vi "erForceRobotControl.vi"(8 "error in (no error)":errorcluster, 10 "robots":T1[](array[typedef]), 11 "Communication in":refnum<class "Communication.lvclass">) -> (0 "error out":errorcluster, 2 "robotControl":u8[](array[numeric]), 3 "Communication out":refnum<class "Communication.lvclass">)   [LabVIEW 2023, in "Communication.lvclass"]
uses:
  Communication.lvclass
  Convert AI Robot to Robot Command Folder/grSim/grSim Robot Command.ctl
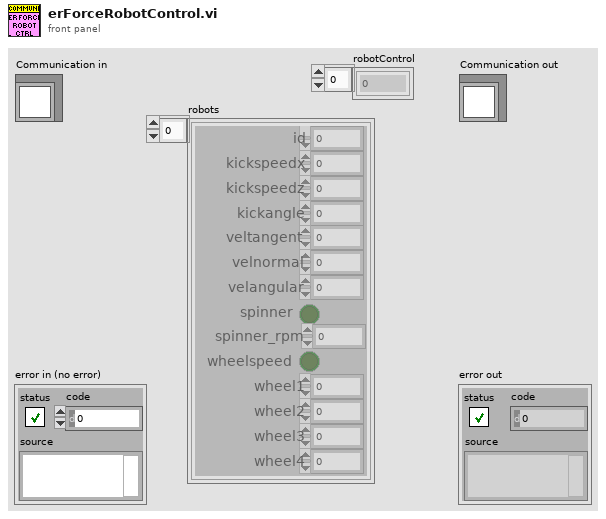
[diagram p1: front panel]
types:
  T1 = typedef "grSim Robot Command.ctl" = cluster{"id":u32, "kickspeedx":sgl, "kickspeedz":sgl, "veltangent":sgl, "velnormal":sgl, "velangular":sgl, "spinner":bool, "wheelspeed":bool, "wheel1":sgl, "wheel2":sgl, "wheel3":sgl, "wheel4":sgl, "kickangle":sgl, "spinner_rpm":sgl}
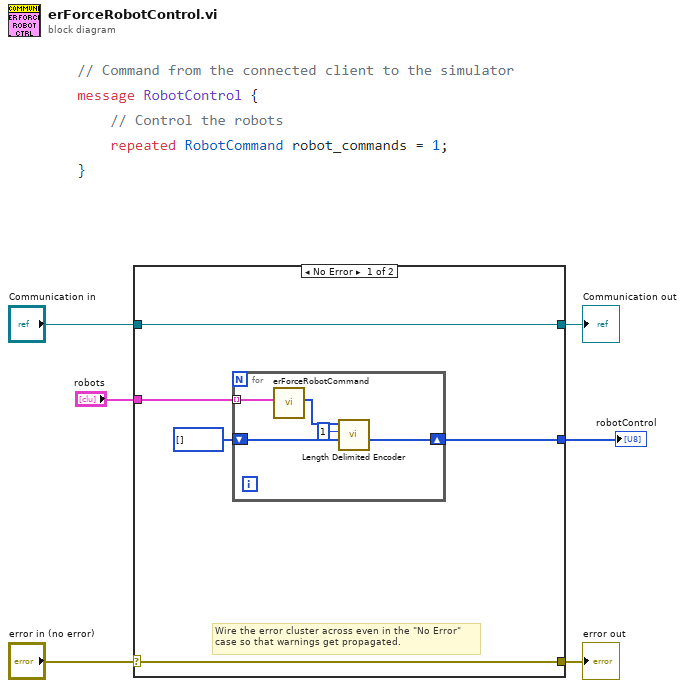
[diagram p0: block diagram]
diagram:
  n1 = case shown="No Error" "error in (no error)" {
    selector: "error in (no error)" -> [w10 w18]
    tunnel: [w10 w18] -> w5
    tunnel: [w11 w17] -> w3
    tunnel: "Communication in" -> [w11 w17]
    tunnel: [w9 _] -> w2
    tunnel: "robots" -> [w8 _]
    frame No Error {
      # "Wire the error cluster across even in the \"No Error\"\ncase so that warnings get propagated."
      n2 = for {
        shift-right: [w15] -> w9
        shift-left: u8[] [] ("Array") -> [w14]
        tunnel: w8 -> [w12] mode=indexing
        n3 = call "erForceRobotCommand.vi"("robot"=w12) -> ("robotCommandArray out"=w16:u8[])  [unwired: 8 in, 2 out]
        n4 = call "Length Delimited Encoder.vi"("Original Array In"=w14, "Key"=u32 1, "Array In to be added"=w16) -> ("Array"=w15:u8[])  [unwired: 8 in]
      }
    }
    frame Error {
    }
  }
  "error out" <- w5
  "Communication out" <- w3
  "robotControl" <- w2
